vi "Rollback Transaction.vi"(8 "error in":errorcluster, 11 "DB-ADO in":refnum<class "DB-ADO.lvclass">) -> (0 "error out":errorcluster, 3 "DB-ADO out":refnum<class "DB-ADO.lvclass">)   [LabVIEW 2022 SP3, in "hse-db-ado.lvlib" / "DB-ADO.lvclass"]
doc: "Rollback the active transaction.\n\n____\nHAMPEL SOFTWARE ENGINEERING v1.4.0 (2023-12-19 09:52)"
uses:
  DB-ADO.lvclass
  DB-ADO.lvclass/DB-ADO.ctl
  ADO-DB-Drivers/ADO-DB-Driver.lvlib
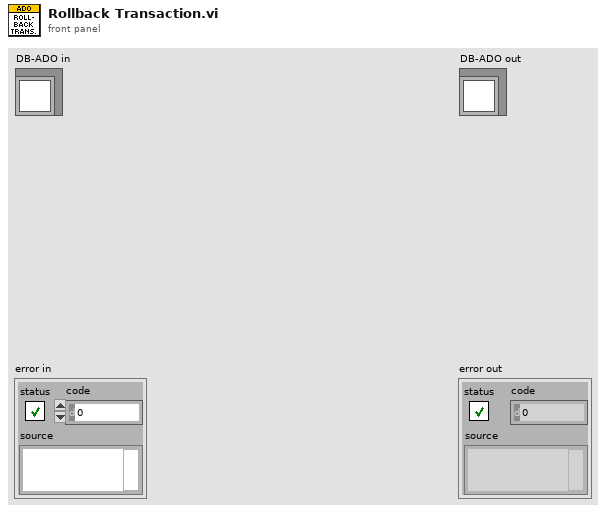
[diagram p1: front panel]
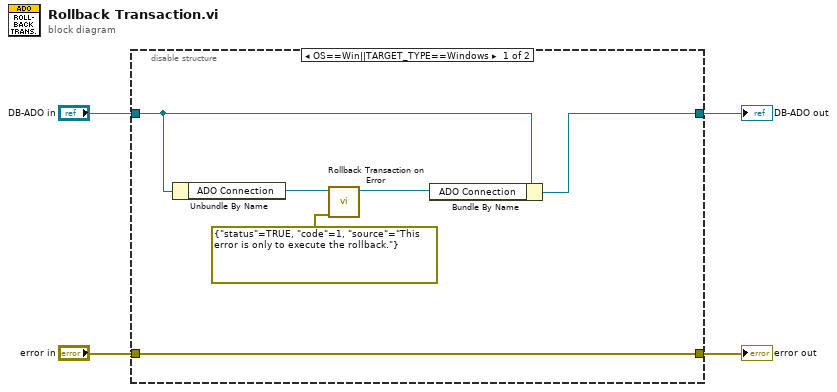
[diagram p0: block diagram]
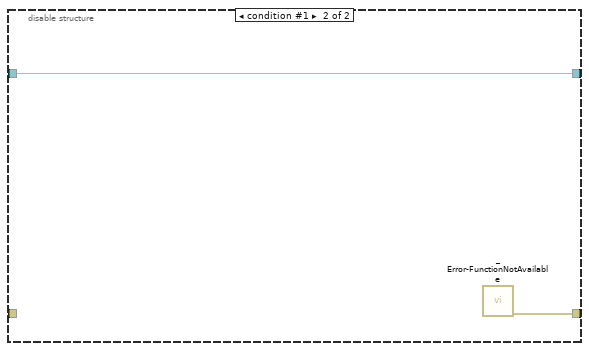
[diagram p2: hidden frame]
diagram:
  n1 = disable-structure shown="OS==Win||TARGET_TYPE==Windows" {
    disable-tunnel: "DB-ADO in" -> [w10 w12]
    disable-tunnel: [w9 w12] -> w1
    disable-tunnel: "error in" -> [w6 _]
    disable-tunnel: [w6 w11] -> w3
    frame condition #0 (active) {
      n2 = Unbundle By Name(w10) -> ("ADO Connection"=w8:refnum<k7>)
      n3 = call "Rollback Transaction on Error.vi"("error in"=errorcluster {"status"=TRUE, "code"=1, "source"="This error is only to execute the rollback."}, "Connection In"=w8) -> ("Connection Out"=w7:refnum<k7>)  [unwired: 7 in, 1 out]
      n4 = Bundle By Name(cluster=w10, "ADO Connection"=w7) -> (w9:refnum<class "DB-ADO.lvclass">)
    }
    frame condition #1 {
      n5 = call "_Error-FunctionNotAvailable.vi"() -> ("error out"=w11:errorcluster)  [unwired: 11 in]
    }
  }
  "error out" <- w3
  "DB-ADO out" <- w1
